vi "read TDI table.vi"() -> ()   [LabVIEW 2023]
uses:
  gfitsio.lvlib
  cfitsio-hdutypes.ctl
  gfitsio-read-column-i16-1d.vi
  cfitsio-bitpix.ctl
  gfitsio-write-image-subset-i32-2d.vi
panel:
  out "new picture":picture
  out "error out":errorcluster
  out "header 2":string[](array[string])
  out "header":string[](array[string])
  out "comment":string
  out "value":string
  out "nelements":i32
  in  "Stop Button":bool
  out "number of rows":i32
  out "x+1":i32
  out "logical AND":bool
  out "Data":i16[][](array[numeric]) caption="1A        1B         2A        2B         3A        3B          4A         4B         5A        5B         6A         6B         7A        7B        8A         8B        9A        9B         10A      10B      11A       11B      12A      12B       13A      13B      14A      14B      15A       15B     16A       16B" format="%04x"
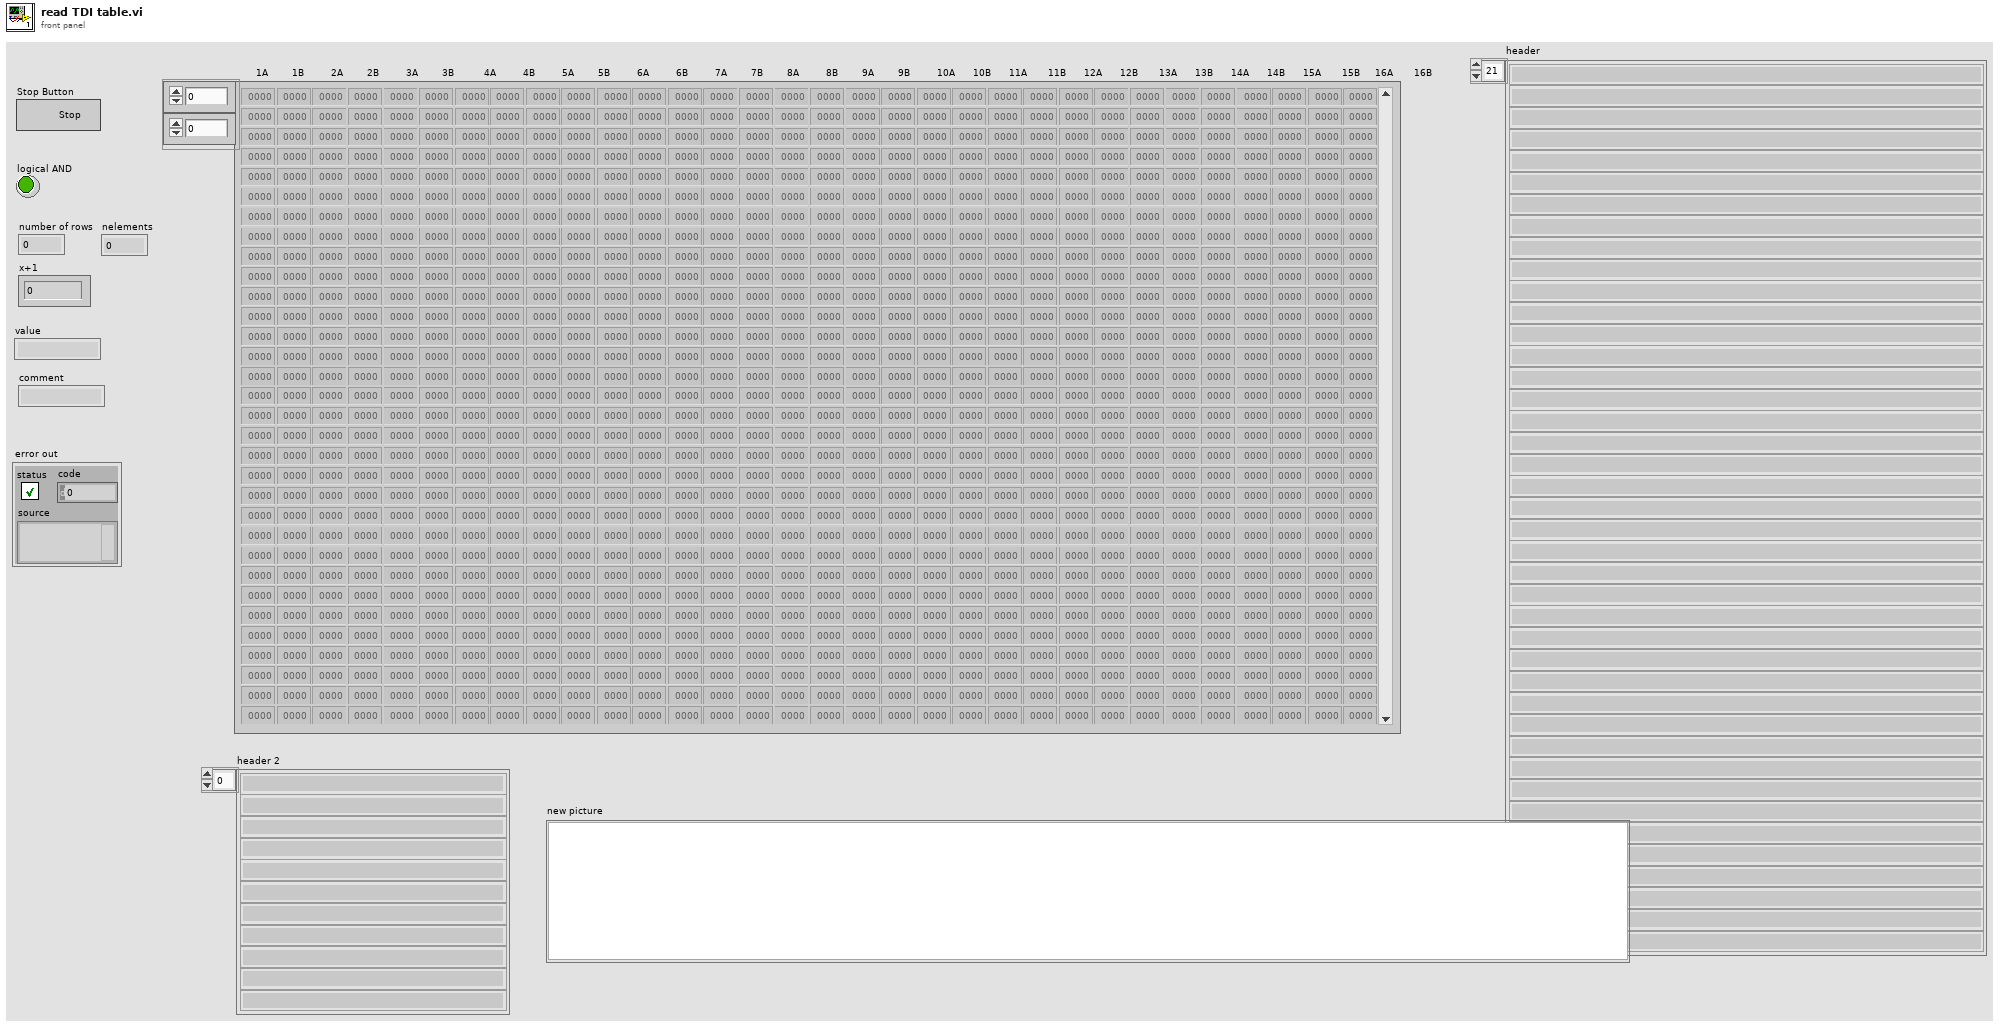
[diagram p1: front panel]
types:
  T1 = typedef "gfitsio.lvlib/cfitsio-bitpix.ctl" = i32
  T2 = typedef "gfitsio.lvlib/cfitsio-hdutypes.ctl" = i32
  T3 = typedef "gfitsio.lvlib/gfitsio-refnum.ctl" = refnum<k1>
  T4 = typedef "imagedata.ctl" = cluster{"image type":i32, "image depth":i32, "image":u8[], "mask":u8[], "colors":u32[], "Rectangle":cluster{"left":i16, "top":i16, "right":i16, "bottom":i16}}
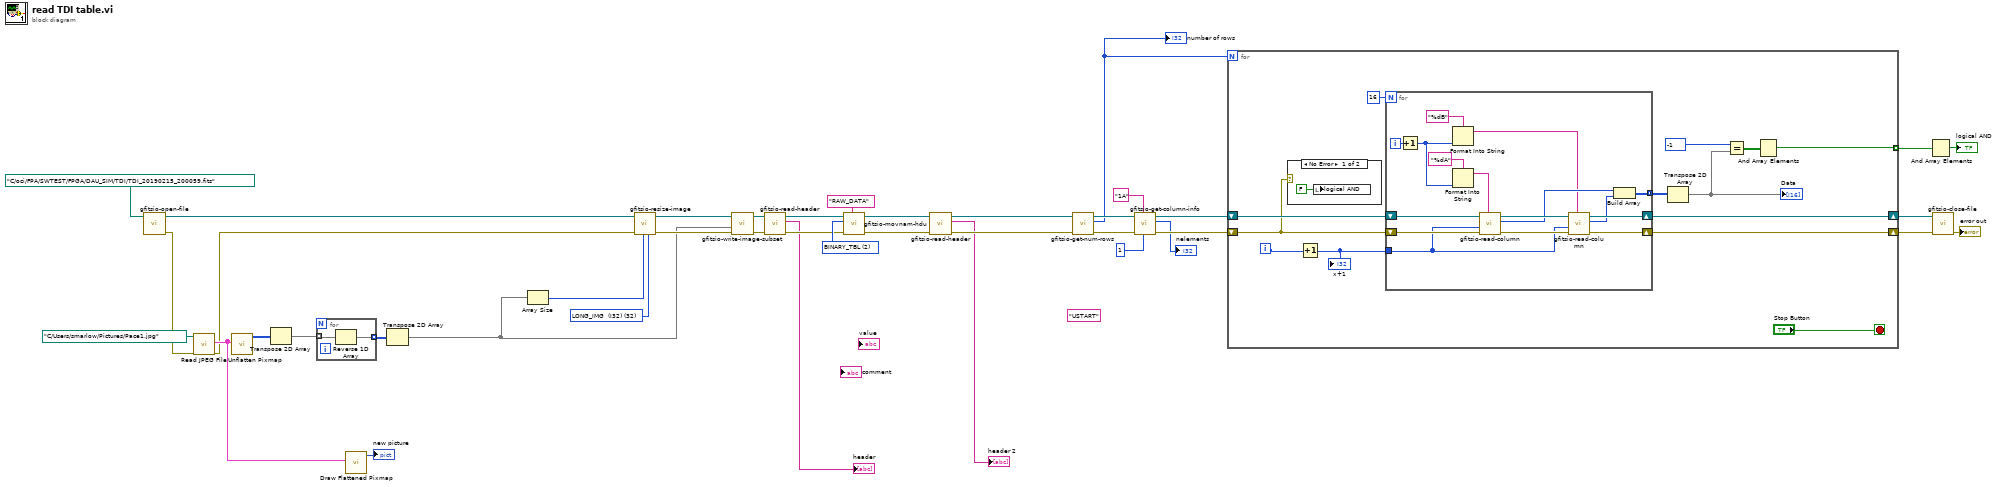
[diagram p0: block diagram]
diagram:
  w10 = T1 32 items=["<invalid type>"=0, "BYTE_IMG  (U8)"=8, "SHORT_IMG  (I16)"=16, "USHORT_IMG  (U16)"=20, "LONG_IMG  (I32)"=32, "ULONG_IMG  (U32)"=40, "FLOAT_IMG  (SGL)"=-32, "DOUBLE_IMG  (DBL)"=-64] ("image data type")
  (unwired) "USTART" ("keyname")
  w37 = T2 2 items=["ANY_HDU"=-1, "IMAGE_HDU"=0, "ASCII_TBL"=1, "BINARY_TBL"=2] ("hdutype (ANY_HDU)")
  n1 = call "gfitsio-open-file.vi"("path"=path "C:/oci/FPA/SWTEST/FPGA/DAU_SIM/TDI/TDI_20190215_200059.fits") -> ("error out"=w13:errorcluster, "gfits refnum"=w39:T3)  [unwired: 9 in]
  n2 = call <vilib>:"Read JPEG File.vi"("error in (no error)"=w13, "path to JPEG file"=path "C:/Users/smarlow/Pictures/Pace1.jpg" ("path to PNG file")) -> ("error out"=w6:errorcluster, "image data"=w9:T4)  [unwired: 7 in, 1 out]
  n3 = call <vilib>:"Unflatten Pixmap.vi"("image data"=w9) -> ("24-bit pixmap"=w4:u32[][])  [unwired: 4 in, 6 out]
  n4 = Transpose 2D Array(2D array=w4) -> (transposed array=w3:u32[][])
  n5 = for {
    tunnel: w3 -> [w42] mode=indexing
    tunnel: [w41] -> w7 mode=indexing
    n6 = Reverse 1D Array(array=w42) -> (reversed array=w41:u32[])
  }
  n7 = call <vilib>:"Draw Flattened Pixmap.vi"("image data"=w9) -> ("new picture"=→"new picture":picture)  [unwired: 8 in]
  n8 = Transpose 2D Array(2D array=w7) -> (transposed array=w1:u32[][])
  n9 = Array Size(array=w1) -> (size(s)=w2:i32[])
  n10 = call "gfitsio-resize-image.vi"("image data type"=w10, "naxes"=w2, "error in (no error)"=w6, "gfits refnum"=w39) -> ("error out"=w11:errorcluster, "dup gfits refnum"=w5:T3)  [unwired: 6 in]
  n11 = call-poly "gfitsio-write-image-subset.vi"("error in (no error)"=w11, "data"=w1, "gfits refnum"=w5) -> ("error out"=w15:errorcluster, "dup gfits refnum"=w16:T3)  [unwired: 7 in]
  n12 = call "gfitsio-read-header.vi"("error in (no error)"=w15, "gfits refnum"=w16) -> ("error out"=w23:errorcluster, "header"=→"header":string[], "dup gfits refnum"=w24:T3)  [unwired: 7 in]
  n13 = call "gfitsio-movnam-hdu.vi"("extname"="RAW_DATA", "error in (no error)"=w23, "hdutype (ANY_HDU)"=w37, "gfits refnum"=w24) -> ("error out"=w20:errorcluster, "dup gfits refnum"=w21:T3)  [unwired: 6 in]
  n14 = call "gfitsio-read-header.vi"("error in (no error)"=w20, "gfits refnum"=w21) -> ("error out"=w18:errorcluster, "header"=→"header 2":string[], "dup gfits refnum"=w19:T3)  [unwired: 7 in]
  n15 = call "gfitsio-get-num-rows.vi"("error in (no error)"=w18, "gfits refnum"=w19) -> ("error out"=w29:errorcluster, "number of rows"=w31:i32, "dup gfits refnum"=w32:T3)  [unwired: 7 in]
  "number of rows" <- w31
  n16 = call "gfitsio-get-column-info.vi"("row (-1: don't check descriptor)"=1, "column"="1A", "error in (no error)"=w29, "gfits refnum"=w32) -> ("error out"=w28:errorcluster, "nelements"=→"nelements":i32, "dup gfits refnum"=w30:T3)  [unwired: 2 in, 3 out]
  n17 = for {
    N: w31 -> [_]
    shift-right: [w53] -> w36
    shift-left: w30 -> [w55]
    shift-right: [w52] -> w35
    shift-left: w28 -> [w54]
    tunnel: [w44] -> w34 mode=indexing
    i -> [w46]
    stop <- "Stop Button" stop-if-true
    n18 = case shown="No Error" w54 {
      frame No Error {
        n19 = local write "logical AND"(FALSE ("logical AND")) -> ()
      }
      frame Error {
      }
    }
    n20 = Increment(x=w46) -> (x+1=w45:i32)
    "x+1" <- w45
    n21 = for {
      N: 16 -> [_]
      shift-right: [w68] -> w53
      shift-left: w55 -> [w72]
      shift-right: [w67] -> w52
      shift-left: w54 -> [w71]
      tunnel: [w64] -> w50 mode=concatenating
      tunnel: w45 -> [w59]
      i -> [w57]
      n22 = Increment(x=w57) -> (x+1=w63:i32)
      n23 = Format Into String(format string="%dB", w63) -> (resulting string=w58:string)  [unwired: 2 in, 1 out]
      n24 = Format Into String(format string="%dA", w63) -> (resulting string=w60:string)  [unwired: 2 in, 1 out]
      n25 = call-poly "gfitsio-read-column.vi"("column"=w60, "error in (no error)"=w71, "row"=w59, "gfits refnum"=w72) -> ("error out"=w69:errorcluster, "data"=w66:i16[], "dup gfits refnum"=w70:T3)  [unwired: 5 in]
      n26 = call-poly "gfitsio-read-column.vi"("column"=w58, "error in (no error)"=w69, "row"=w59, "gfits refnum"=w70) -> ("error out"=w67:errorcluster, "data"=w65:i16[], "dup gfits refnum"=w68:T3)  [unwired: 5 in]
      n27 = Build Array(w66, w65) -> (w64:i16[][])
    }
    n28 = Transpose 2D Array(2D array=w50) -> (transposed array=w49:i16[][])
    "Data" <- w49
    n29 = Equal?(x=i16 -1, y=w49) -> (x = y?=w47:bool[][])
    n30 = And Array Elements(Boolean array=w47) -> (logical AND=w44:bool)
  }
  n31 = And Array Elements(Boolean array=w34) -> (logical AND=→"logical AND":bool)
  n32 = call "gfitsio-close-file.vi"("error in (no error)"=w35, "gfits refnum"=w36) -> ("error out"=→"error out":errorcluster)  [unwired: 8 in, 1 out]
